vi "Write Channel Map.vi"(8 "error in (no error)":errorcluster, 10 "Channel Map":map{string, refnum<class "CIFChannels.lvclass">}(c390), 11 "CIFChannelMng in":refnum<class "CIFChannelMng.lvclass">) -> (0 "error out":errorcluster, 3 "CIFChannelMng out":refnum<class "CIFChannelMng.lvclass">)   [LabVIEW 2021, in "CIFChannelMng.lvclass"]
uses:
  CIFChannelMng.lvclass
  CIFChannelMng.lvclass/CIFChannelMng.ctl
  CIFChannels/CIFChannels.lvclass
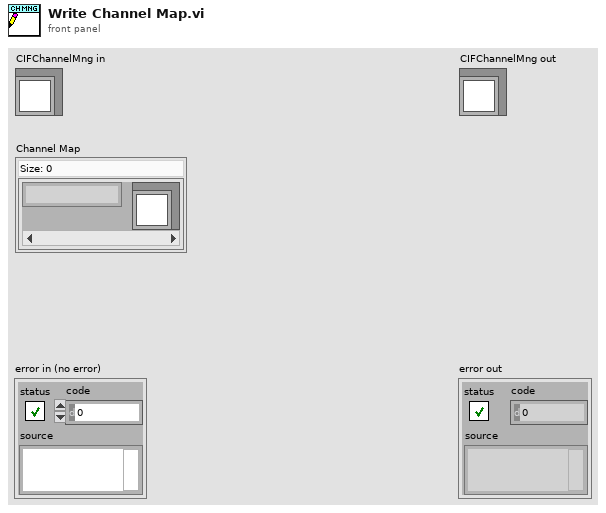
[diagram p1: front panel]
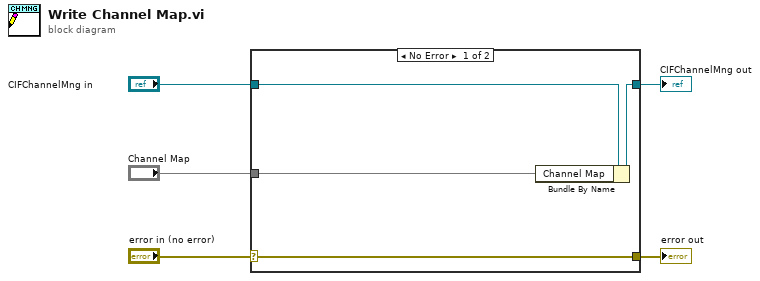
[diagram p0: block diagram]
diagram:
  n1 = case shown="No Error" "error in (no error)" {
    selector: "error in (no error)" -> [w9 w10]
    tunnel: [w9 w10] -> w4
    tunnel: [w7 w11] -> w2
    tunnel: "CIFChannelMng in" -> [w8 w11]
    tunnel: "Channel Map" -> [w6 _]
    frame No Error {
      n2 = Bundle By Name(cluster=w8, "Channel Map"=w6) -> (w7:refnum<class "CIFChannelMng.lvclass">)
    }
    frame Error {
    }
  }
  "error out" <- w4
  "CIFChannelMng out" <- w2
